vi "Configure Test Sequence.vi"(6 "Trigger Link Line (1: Line1)":i32(ring)=1 items=["Line1"=1, "Line2"=2, "Line3"=3, "Line4"=4, "Line5"=5, "Line6"=6], 7 "Control Source (0: Manual)":i32(ring) items=["Manual", "Immediate", "Bus", "External", "Trigger link", "Lid closure"], 8 "error in (no error)":errorcluster, 9 "Test Sequence Type (9: Alternating polarity resistance resistivity)":i32(ring)=9 items=["Diode leakage", "Capacitor leakage", "Cable insulation resistance", "Resistor voltage coefficient", "Surface resistivity", "Volume resistivity", "Surface insulation resistance", "Square wave sweep", "Staircase sweep", "Alternating polarity resistance resistivity"], 10 "Test Sequence Option (0: Abort)":i32(ring) items=["Abort", "Arm"], 11 "VISA resource name":refnum<visa-resource-name>) -> (0 "error out":errorcluster, 3 "VISA resource name out":refnum<visa-resource-name>)   [LabVIEW 2020, in "Keithley 6517.lvlib"]
doc: "Configures test sequence common characteristics, to abort or arm test sequence, configures the test sequence type and the start event. When the start event is trigger link, the link line should be configured as well. \n\nNote: \nThis VI should be called first before configures the settings of all kinds of test sequence.\n\nThis VI is <B>NOT</B> compatible with model <B>6514</B>."
uses:
  <instrlib>/Keithley 6517/Keithley 6517.lvlib
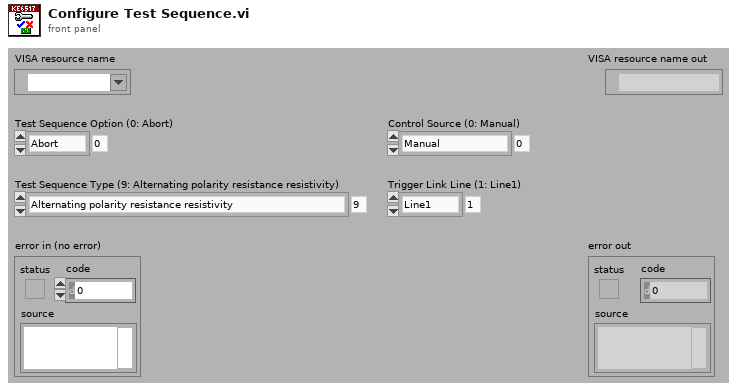
[diagram p1: front panel]
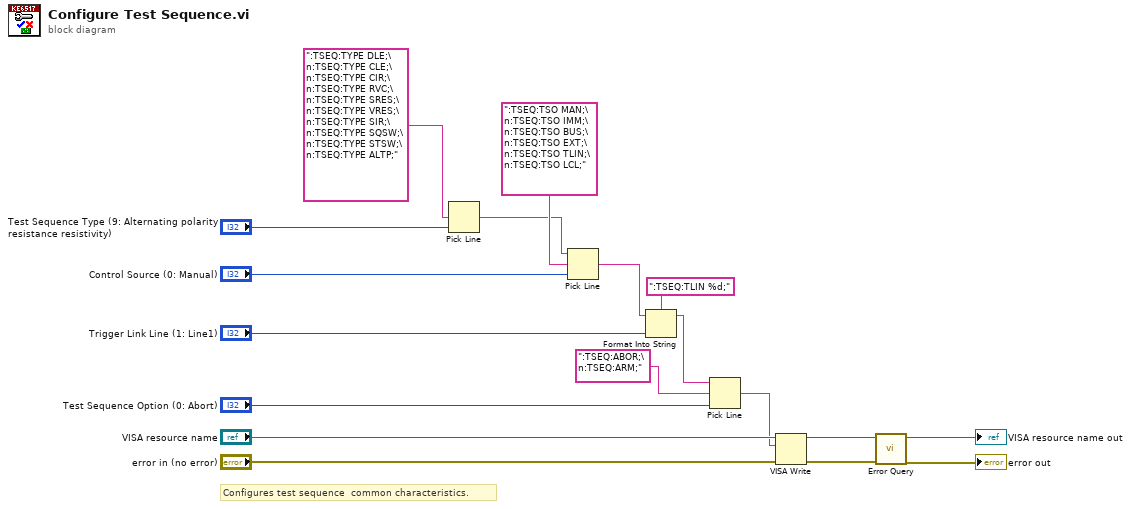
[diagram p0: block diagram]
diagram:
  # "Configures test sequence  common characteristics."
  n1 = Pick Line(multi-line string=":TSEQ:TYPE DLE;\n:TSEQ:TYPE CLE;\n:TSEQ:TYPE CIR;\n:TSEQ:TYPE RVC;\n:TSEQ:TYPE SRES;\n:TSEQ:TYPE VRES;\n:TSEQ:TYPE SIR;\n:TSEQ:TYPE SQSW;\n:TSEQ:TYPE STSW;\n:TSEQ:TYPE ALTP;", line index="Test Sequence Type (9: Alternating polarity resistance resistivity)") -> (output string=w5:string)  [unwired: 1 in]
  n2 = Pick Line(string ("")=w5, multi-line string=":TSEQ:TSO MAN;\n:TSEQ:TSO IMM;\n:TSEQ:TSO BUS;\n:TSEQ:TSO EXT;\n:TSEQ:TSO TLIN;\n:TSEQ:TSO LCL;", line index="Control Source (0: Manual)") -> (output string=w4:string)
  n3 = Format Into String(format string=":TSEQ:TLIN %d;", initial string=w4, "Trigger Link Line (1: Line1)") -> (resulting string=w2:string)  [unwired: 1 in, 1 out]
  n4 = Pick Line(string ("")=w2, multi-line string=":TSEQ:ABOR;\n:TSEQ:ARM;", line index="Test Sequence Option (0: Abort)") -> (output string=w1:string)
  n5 = VISA Write(VISA resource name="VISA resource name", write buffer=w1, error in (no error)="error in (no error)") -> (VISA resource name out=w14:refnum<visa-resource-name>, error out=w13:errorcluster)  [unwired: 1 out]
  n6 = call <instrlib>:"Error Query.vi"("error in (no error)"=w13, "VISA resource name"=w14) -> ("error out"=→"error out":errorcluster, "VISA resource name out"=→"VISA resource name out":refnum<visa-resource-name>)  [unwired: 6 in, 2 out]
